vi "thermometer.vi"(8 "error in (no error)":errorcluster, 10 "Lower Bound":dbl, 11 "Upper Bound":dbl) -> (0 "error out":errorcluster, 3 "random temp":dbl)   [LabVIEW 2014]
uses:
  <vilib>/Utility/error.llb/DialogType.ctl
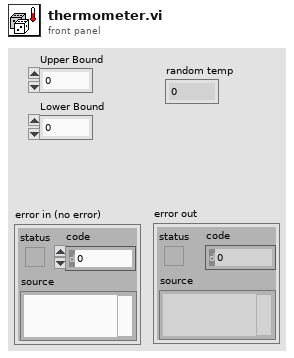
[diagram p1: front panel]
types:
  T1 = typedef "DialogType.ctl" = u16
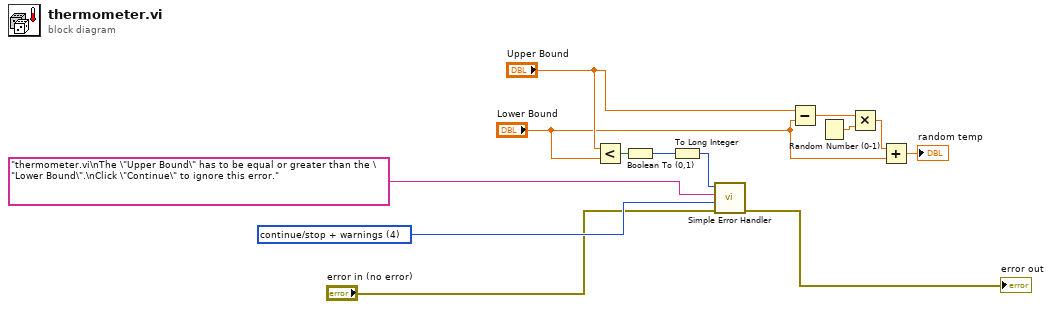
[diagram p0: block diagram]
diagram:
  w9 = T1 4 items=["no dialog", "OK message", "continue or stop message", "OK message + warnings", "continue/stop + warnings"] ("type of dialog (OK msg:1)")
  n1 = Less?(x="Upper Bound", y="Lower Bound") -> (x < y?=w6:bool)
  n2 = Boolean To (0,1)(Boolean=w6) -> (0, 1=w5:i16)
  n3 = To Long Integer(number=w5) -> (32bit integer=w4:i32)
  n4 = call <vilib>:"Simple Error Handler.vi"("error code (no error:0)"=w4, "error source (\" \")"="thermometer.vi\nThe \"Upper Bound\" has to be equal or greater than the \"Lower Bound\".\nClick \"Continue\" to ignore this error." ("message"), "type of dialog (OK msg:1)"=w9, "error in (no error)"="error in (no error)") -> ("error out"=→"error out":errorcluster)  [unwired: 1 in, 4 out]
  n5 = Subtract(x="Upper Bound", y="Lower Bound") -> (x-y=w13:dbl)
  n6 = Random Number (0-1)() -> (number: 0 to 1=w12:dbl)
  n7 = Multiply(x=w13, y=w12) -> (x*y=w11:dbl)
  n8 = Add(x=w11, y="Lower Bound") -> (x+y=→"random temp":dbl)
